vi "Target - To More Specific Class.vi"() -> ()   [LabVIEW 2023]
doc: "This VI is used by the To More Specific Class.vi example."
panel:
  in  "Tree 2":string(tree)
  in  "Multicolumn Listbox 2":i32(listbox)
  in  "Listbox 2":i32(listbox)
  in  "Tree":string(tree)
  in  "Multicolumn Listbox":i32(listbox)
  in  "Listbox":i32(listbox)
  # "This VI is used by the To More Specific Class.vi example."
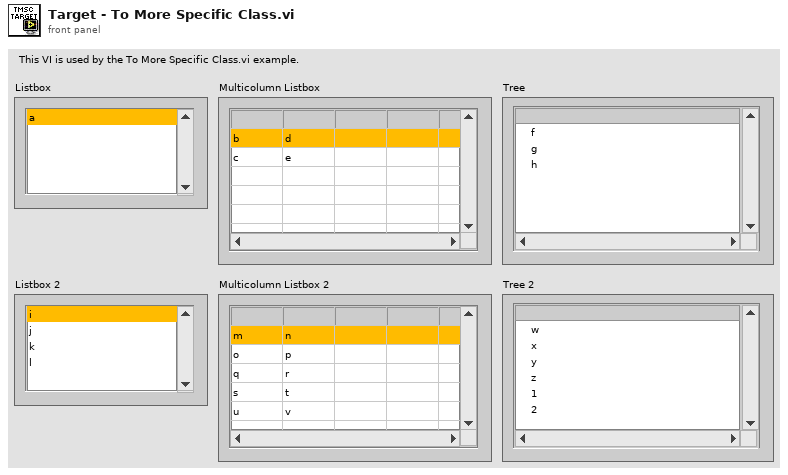
[diagram p1: front panel]
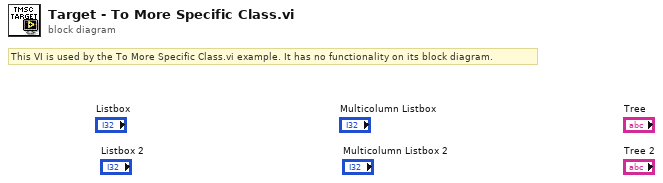
[diagram p0: block diagram]
diagram:
  # "This VI is used by the To More Specific Class.vi example. It has no functionality on its block diagram."
